vi "Load Framework.vi"(8 "error in (no error)":errorcluster, 11 "Application Refs":T1) -> (0 "error out":errorcluster, 3 "Application Data out":T1)   [LabVIEW 2017, in "DSF Data Viewer.lvlib"]
uses:
  DSF Data Viewer.lvlib
  Application Data.ctl
  <vilib>/NI/Memory Manager/Classes/Pointer/Pointer.lvclass
  Builds/Data Sharing Framework/Current/Core/DSF Core.lvlibp/Engine/Classes/Framework/Framework.lvclass
  Buffer Reader/Buffer Data.ctl
  Builds/Data Sharing Framework/Current/Core/DSF Core.lvlibp/Engine/Classes/Buffer/Buffer.lvclass
  Builds/Data Sharing Framework/Current/Core/DSF Core.lvlibp/Engine/Classes/Transfer Group Status/Transfer Group Status.lvclass
  Item Tree/Add Plugin with Children.vi
  Item Tree/Create New Tree Item.vi
  Item Tree/Add Transfer Group with Children.vi
  Item Tree/Add Buffer Data to Variant.vi
  Item Tree/Add Transfer.vi
  Item Tree/Add Buffers.vi
  Item Tree/Add Item to Tree.vi
  Builds/Data Sharing Framework/Current/Core/DSF Core.lvlibp/Engine/Classes/Buffer/Get String Buffer.vi
  Builds/Data Sharing Framework/Current/Core/DSF Core.lvlibp/Engine/Classes/Buffer/Get Async Buffer.vi
  Builds/Data Sharing Framework/Current/Core/DSF Core.lvlibp/Engine/Classes/Buffer/Get Inline Buffer.vi
  Builds/Data Sharing Framework/Current/Core/DSF Core.lvlibp/Engine/Classes/Transfer/Get Buffers.vi
  Builds/Data Sharing Framework/Current/Core/DSF Core.lvlibp/Engine/Classes/Transfer/Get Name.vi
  Builds/Data Sharing Framework/Current/Core/DSF Core.lvlibp/Engine/Classes/Timing/Get Decimation.vi
  Builds/Data Sharing Framework/Current/Core/DSF Core.lvlibp/Engine/Classes/Transfer Group/Get Inline.vi
  Builds/Data Sharing Framework/Current/Core/DSF Core.lvlibp/Engine/Classes/Transfer Group/Get Transfers.vi
  Builds/Data Sharing Framework/Current/Core/DSF Core.lvlibp/Engine/Classes/Transfer Group/Get Status.vi
  Builds/Data Sharing Framework/Current/Core/DSF Core.lvlibp/Engine/Classes/Transfer Group/Get Timing.vi
  Builds/Data Sharing Framework/Current/Core/DSF Core.lvlibp/Engine/Classes/Transfer Group/Get Name.vi
  Builds/Data Sharing Framework/Current/Core/DSF Core.lvlibp/Engine/Classes/Plugin/Get Name.vi
  Builds/Data Sharing Framework/Current/Core/DSF Core.lvlibp/Engine/Classes/Plugin/Get Async Rx Transfer Groups.vi
  Builds/Data Sharing Framework/Current/Core/DSF Core.lvlibp/Engine/Classes/Plugin/Get Async Tx Transfer Groups.vi
  Builds/Data Sharing Framework/Current/Core/DSF Core.lvlibp/Engine/Classes/Plugin/Get Inline Rx Transfer Groups.vi
  Builds/Data Sharing Framework/Current/Core/DSF Core.lvlibp/Engine/Classes/Plugin/Get Inline Tx Transfer Groups.vi
  Builds/Data Sharing Framework/Current/Core/DSF Core.lvlibp/Engine/Classes/Plugin/Get Buffers.vi
  Builds/Data Sharing Framework/Current/Core/DSF Core.lvlibp/Engine/Classes/Plugin/Get Timing.vi
  Builds/Data Sharing Framework/Current/Core/DSF Core.lvlibp/Engine/Classes/Framework/Get Async Plugins.vi
  Builds/Data Sharing Framework/Current/Core/DSF Core.lvlibp/Engine/Classes/Framework/Get Inline Plugins.vi
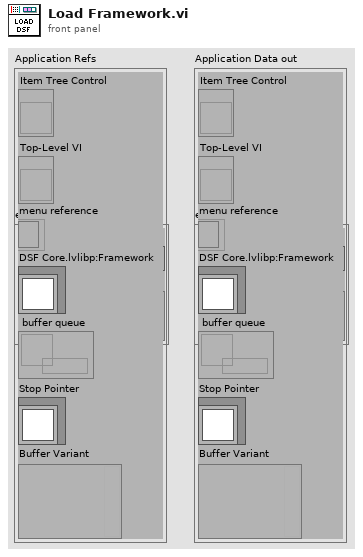
[diagram p1: front panel]
types:
  T1 = typedef "DSF Data Viewer.lvlib/Application Data.ctl" = cluster{"Item Tree Control":refnum<vi>, "Top-Level VI":refnum<vi>, "menu reference":refnum<k9>, "DSF Core.lvlibp:Framework":refnum<class "Framework.lvclass">, "buffer queue":refnum<queue>, "Stop Pointer":refnum<class "Pointer.lvclass">, "Buffer Variant":variant}
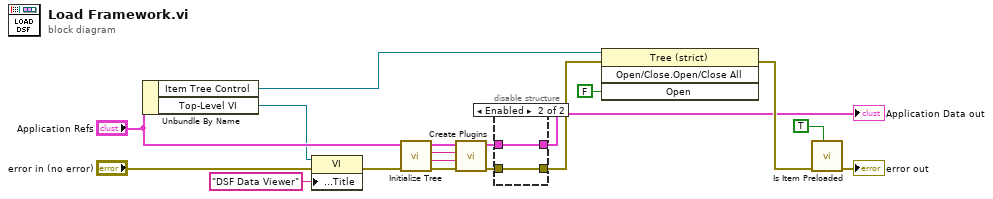
[diagram p0: block diagram]
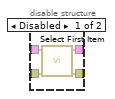
[diagram p2: hidden frame]
diagram:
  n1 = Unbundle By Name("Application Refs") -> ("Item Tree Control"=w5:refnum<vi>, "Top-Level VI"=w16:refnum<vi>)
  n2 = property class="VI"(reference=w16, error in="error in (no error)", "Front Panel.Title"="DSF Data Viewer" ("Front Panel Window:Title")) -> (error out=w18:errorcluster)  [unwired: 1 out]
  n3 = call "Initialize Tree.vi"("error in (no error)"=w18, "Application Data in"="Application Refs") -> ("error out"=w10:errorcluster, "async plugins tag"=w8:string, "inline plugins tag"=w9:string, "Application Data out"=w11:T1)  [unwired: 6 in]
  n4 = call "Create Plugins.vi"("error in (no error)"=w10, "async plugins tag"=w8, "inline plugins tag"=w9, "Application Data In"=w11) -> ("error out"=w6:errorcluster, "Application Data out"=w7:T1)  [unwired: 6 in]
  n5 = disable-structure shown="Enabled" {
    disable-tunnel: w7 -> [w22 w23]
    disable-tunnel: w6 -> [w21 w24]
    disable-tunnel: [w20 w24] -> w3
    disable-tunnel: [w19 w23] -> w1
    frame Disabled {
      n6 = call "Select First Item.vi"("error in (no error)"=w21, "Application Data in"=w22) -> ("error out"=w20:errorcluster, "Application Data out"=w19:T1)  [unwired: 8 in]
    }
    frame Enabled {
    }
  }
  "Application Data out" <- w1
  n7 = invoke class="Tree (strict)" method="Open/Close.Open/Close All"(reference=w5, error in=w3, "Open"=FALSE ("Open?")) -> (error out=w2:errorcluster)  [unwired: 1 in, 3 out]
  n8 = call "Is Item Preloaded"("clear entries"=TRUE, "error in (no error)"=w2) -> ("error out"=→"error out":errorcluster)  [unwired: 7 in, 2 out]
